vi "Write String Array (1D).vi"(6 "error in":errorcluster, 8 "Value":string[](array[string]), 9 "String Array (1D) Ref in":refnum<vi>) -> (0 "error out":errorcluster, 3 "String Array (1D) Ref out":refnum<vi>)   [LabVIEW 2020, in "G-Unicode.lvlib"]
uses:
  G-Unicode.lvlib
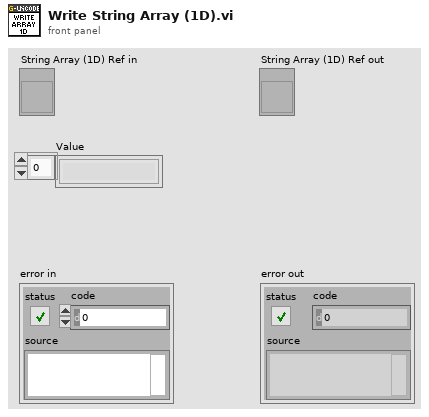
[diagram p1: front panel]
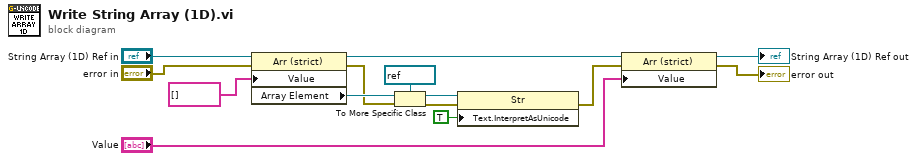
[diagram p0: block diagram]
diagram:
  n1 = property class="Arr (strict)"(reference="String Array (1D) Ref in", error in="error in", "Value"=string[] []) -> (reference out=w5:refnum<vi>, error out=w12:errorcluster, "Array Element"=w13:refnum<vi>)
  n2 = To More Specific Class(target class=refnum<vi> refnum ("String"), reference=w13, error in=w12) -> (specific class reference=w11:refnum<vi>, error out=w8:errorcluster)
  n3 = property class="Str"(reference=w11, error in=w8, "Text.InterpretAsUnicode"=TRUE ("Text.Interpret As Unicode")) -> (error out=w3:errorcluster)  [unwired: 1 out]
  n4 = property class="Arr (strict)"(reference=w5, error in=w3, "Value"="Value") -> (reference out=→"String Array (1D) Ref out":refnum<vi>, error out=→"error out":errorcluster)
